vi "_FPGA_Driver_sub_AD5648_32bit_Encode.vi"(9 "data_U14":fxp<+,14,14>, 10 "address_U4":fxp<+,4,4>, 11 "cmd":fxp<+,4,4>) -> (2 "Data_out":bool[](array[boolean]))   [LabVIEW 2018]
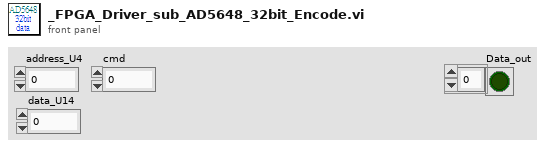
[diagram p1: front panel]
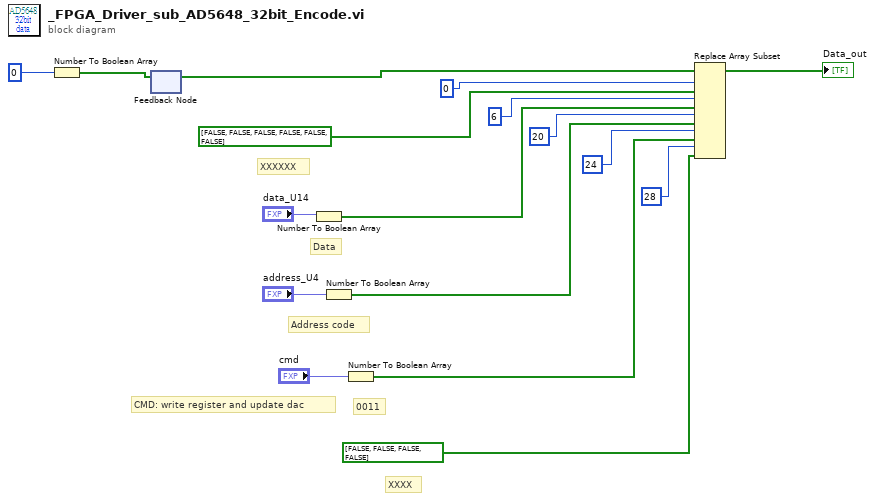
[diagram p0: block diagram]
diagram:
  # "XXXXXX"
  # "Data"
  # "Address code"
  # "CMD: write register and update dac"
  # "0011"
  # "XXXX"
  n1 = Number To Boolean Array(number=u32 0) -> (Boolean array=w14:bool[])
  n2 = feedback-in #1(w14) -> ()
  n3 = feedback #1() -> (w13:bool[])  [unwired: 1 in]
  n4 = Number To Boolean Array(number="data_U14") -> (Boolean array=w8:bool[])
  n5 = Number To Boolean Array(number="address_U4") -> (Boolean array=w7:bool[])
  n6 = Number To Boolean Array(number="cmd") -> (Boolean array=w1:bool[])
  n7 = Replace Array Subset(array=w13, new element #1=bool[] [FALSE, FALSE, FALSE, FALSE, FALSE, FALSE], index #1=0 ("index"), new element #2=w8, index #2=6 ("index"), new element #3=w7, index #3=20 ("index"), new element #4=w1, index #4=24 ("index"), new element #5=bool[] [FALSE, FALSE, FALSE, FALSE], index #5=28 ("index")) -> (→"Data_out":bool[])
